vi "Parse Variant.vi"(8 "error in":errorcluster, 10 "Data":variant) -> (0 "error out":errorcluster, 1 "Types":T1[](array[typedef]), 2 "Data":string[](array[string]), 3 "Variants":variant[](array[variant]), 4 "Type (Name)":string[](array[string]))   [LabVIEW 2019, in "LV-Data.PGSQL.lvclass"]
uses:
  LV-Data.PGSQL.lvclass
  <vilib>/Utility/Data Type/Type Definitions/Data Type.ctl
  Typedefs/Errors--enum.ctl
  Typedefs/Time.Datatype--enum.ctl
  <vilib>/Utility/Data Type/NI_Data Type.lvlib
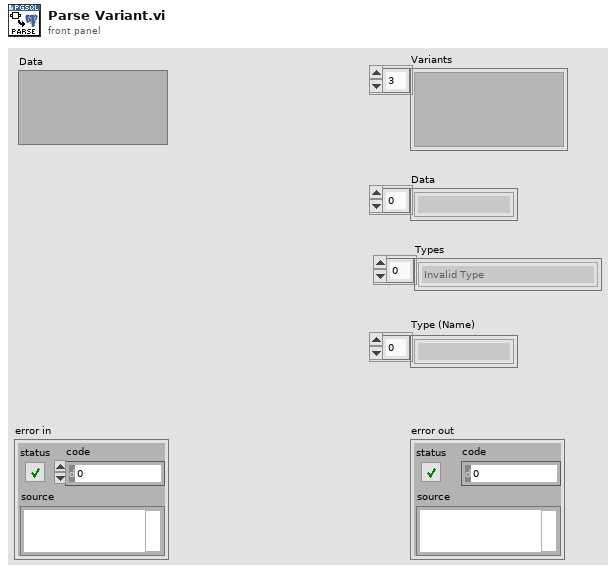
[diagram p1: front panel]
types:
  T1 = typedef "NI_Data Type.lvlib/Data Type.ctl" = enum8{"Invalid Type", "Void", "I8", "I16", "I32", "I64", "U8", "U16", "U32", "U64", "Single Float", "Double Float", "Extended Float", "Single Complex", "Double Complex", "Extended Complex", "Enum U8", "Enum U16", "Enum U32", "Enum U64", "Single Float With Unit", "Double Float With Unit", "Extended Float With Unit", "Single Complex with Unit", "Double Complex with Unit", "Extended Complex with Unit", "Boolean", "String", "Path", "Picture", "Tag", "Array", "Cluster", "Variant", "LV Variant", "Waveform", "Timestamp", "Digital Waveform", "Digital Data", "ExpressData", "Refnum", "External Data", "VI", "Poly VI", "LabVIEW Class Instance", "Fixed Point", "Set Collection", "Map Collection"}
  T2 = typedef "LV-Data.PGSQL.lvclass/Errors--enum.ctl" = enum16{"0: None", "5005: Path Type Not Supported", "5006: Number of Variables", "5007: Number of data points", "5008: Cannot write two data points", "5030: Start and End Times Identical", "5031: Input is not wholly", "5032: Undefined Timestamps", "5033: Bad path or paths", "5040: Invalid Instrument Name", "5050: Column can only hold string", "5051: Column can only hold bool", "5052: Column can only hold double", "5053: Column can only hold int"}
  T3 = typedef "LV-Data.PGSQL.lvclass/Time.Datatype--enum.ctl" = enum16{"timestamp without time zone", "timestamp with time zone"}
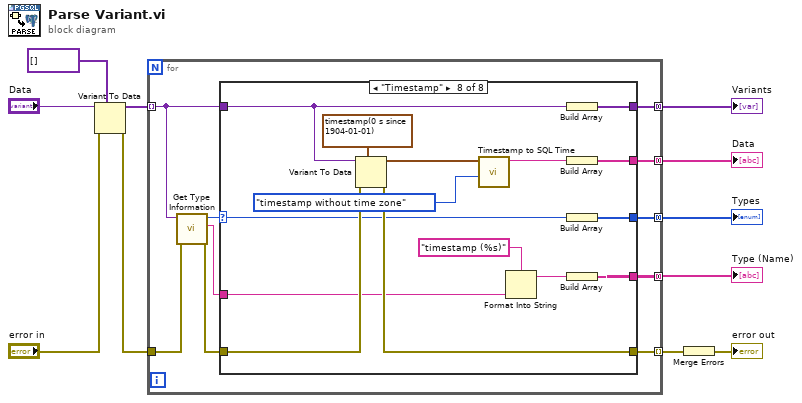
[diagram p0: block diagram]
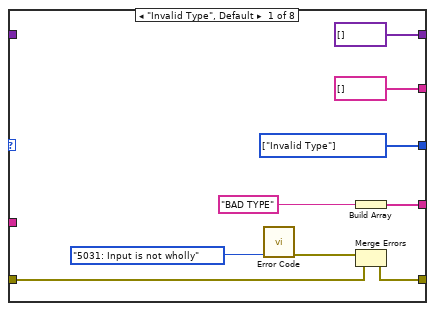
[diagram p2: hidden frame]
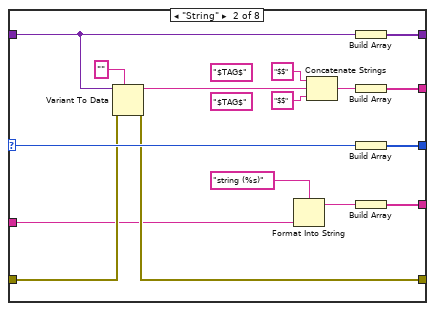
[diagram p3: hidden frame]
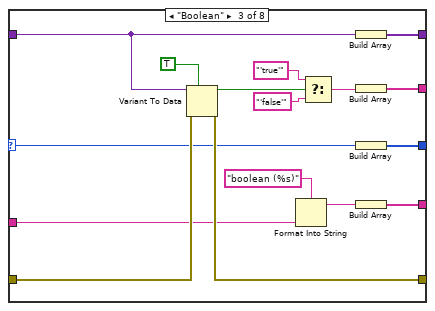
[diagram p4: hidden frame]
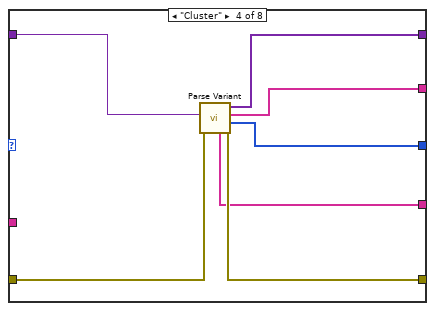
[diagram p5: hidden frame]
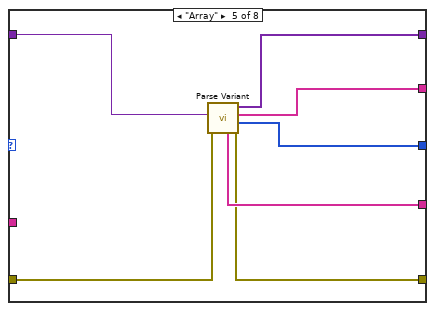
[diagram p6: hidden frame]
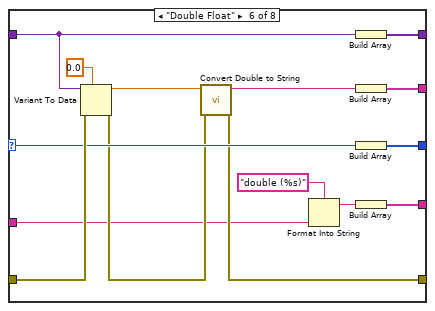
[diagram p7: hidden frame]
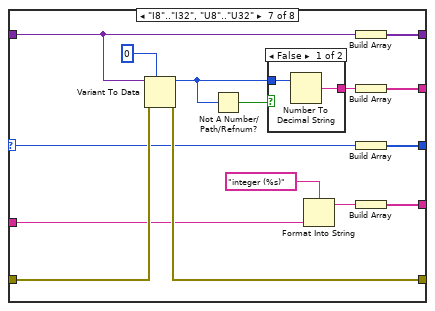
[diagram p8: hidden frame]
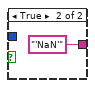
[diagram p9: hidden frame]
diagram:
  n1 = Variant To Data(error in="error in", type=variant[] [] ("Variants"), Variant="Data") -> (data=w2:variant[], error out=w3:errorcluster)
  n2 = for {
    tunnel: w2 -> [w16] mode=indexing
    tunnel: [w20] -> w11 mode=concatenating
    tunnel: [w19] -> w10 mode=concatenating
    tunnel: [w18] -> w9 mode=concatenating
    tunnel: [w13] -> w7 mode=indexing
    tunnel: w3 -> [w15]
    tunnel: [w17] -> w6 mode=concatenating
    n3 = call <vilib>:"Get Type Information.vi"("error in (no error)"=w15, "variant"=w16) -> ("error out"=w14:errorcluster, "name"=w12:string, "type"=w21:T1)  [unwired: 5 in, 2 out]
    n4 = case shown="\"Timestamp\"" w21 {
      selector: w21 -> [_ w36 w50 _ _ w83 w98 w118]
      tunnel: w16 -> [_ w39 w55 w69 w76 w86 w95 w117]
      tunnel: [string[] [] ("Strings") w41 w57 w64 w75 w89 w103 w122] -> w19
      tunnel: [w28 w40 w56 w65 w70 w90 w105 w124] -> w20
      tunnel: [variant[] [] ("Variants") w38 w54 w63 w71 w87 w104 w123] -> w18
      tunnel: [w27 w37 w53 w66 w74 w85 w101 w121] -> w17
      tunnel: w14 -> [w25 w35 w52 w68 w73 w84 w100 w120]
      tunnel: [w24 w34 w51 w67 w72 w80 w99 w119] -> w13
      tunnel: w12 -> [_ w32 w49 _ _ w78 w92 w112]
      frame "Invalid Type", Default {
        w28 = T1[] [enum."Invalid Type"] items=["Invalid Type", "Void", "I8", "I16", "I32", "I64", "U8", "U16", "U32", "U64", "Single Float", "Double Float", "Extended Float", "Single Complex", "Double Complex", "Extended Complex", "Enum U8", "Enum U16", "Enum U32", "Enum U64", "Single Float With Unit", "Double Float With Unit", "Extended Float With Unit", "Single Complex with Unit", "Double Complex with Unit", "Extended Complex with Unit", "Boolean", "String", "Path", "Picture", "Tag", "Array", "Cluster", "Variant", "LV Variant", "Waveform", "Timestamp", "Digital Waveform", "Digital Data", "ExpressData", "Refnum", "External Data", "VI", "Poly VI", "LabVIEW Class Instance", "Fixed Point", "Set Collection", "Map Collection"] ("Types")
        n5 = call "Error Code.vi"("Error code"=Errors--enum."5031: Input is not wholly") -> ("error out"=w22:errorcluster)  [unwired: 10 in]
        n6 = Build Array("BAD TYPE") -> (w27:string[])
        n7 = Merge Errors(w22, w25) -> (w24:errorcluster)
      }
      frame "String" {
        (unwired) "$TAG$" ("string")
        (unwired) "$TAG$" ("string")
        n8 = Variant To Data(error in=w35, type="", Variant=w39) -> (data=w45:string, error out=w34:errorcluster)
        n9 = Format Into String(format string="string (%s)", w32) -> (resulting string=w31:string)  [unwired: 2 in, 1 out]
        n10 = Concatenate Strings("$$" ("string"), w45, "$$" ("string")) -> (w42:string)
        n11 = Build Array(w39) -> (w38:variant[])
        n12 = Build Array(w42) -> (w41:string[])
        n13 = Build Array(w36) -> (w40:T1[])
        n14 = Build Array(w31) -> (w37:string[])
      }
      frame "Boolean" {
        n15 = Variant To Data(error in=w52, type=TRUE, Variant=w55) -> (data=w61:bool, error out=w51:errorcluster)
        n16 = Format Into String(format string="boolean (%s)", w49) -> (resulting string=w48:string)  [unwired: 2 in, 1 out]
        n17 = Select(t="'true'", s=w61, f="'false'") -> (s? t:f=w58:string)
        n18 = Build Array(w55) -> (w54:variant[])
        n19 = Build Array(w58) -> (w57:string[])
        n20 = Build Array(w50) -> (w56:T1[])
        n21 = Build Array(w48) -> (w53:string[])
      }
      frame "Cluster" {
        n22 = call "Parse Variant.vi"("error in"=w68, "Data"=w69) -> ("error out"=w67:errorcluster, "Types"=w65:T1[], "Data"=w64:string[], "Variants"=w63:variant[], "Type (Name)"=w66:string[])  [unwired: 5 in]
      }
      frame "Array" {
        n23 = call "Parse Variant.vi"("error in"=w73, "Data"=w76) -> ("error out"=w72:errorcluster, "Types"=w70:T1[], "Data"=w75:string[], "Variants"=w71:variant[], "Type (Name)"=w74:string[])  [unwired: 5 in]
      }
      frame "Double Float" {
        n24 = Variant To Data(error in=w84, type=0.0, Variant=w86) -> (data=w82:dbl, error out=w81:errorcluster)
        n25 = call "Convert Double to String.vi"("error in"=w81, "Numeric"=w82) -> ("error out"=w80:errorcluster, "PGSQL String"=w88:string)  [unwired: 8 in]
        n26 = Format Into String(format string="double (%s)", w78) -> (resulting string=w77:string)  [unwired: 2 in, 1 out]
        n27 = Build Array(w86) -> (w87:variant[])
        n28 = Build Array(w88) -> (w89:string[])
        n29 = Build Array(w83) -> (w90:T1[])
        n30 = Build Array(w77) -> (w85:string[])
      }
      frame "I8".."I32", "U8".."U32" {
        n31 = Variant To Data(error in=w100, type=0, Variant=w95) -> (data=w96:i32, error out=w99:errorcluster)
        n32 = Not A Number/Path/Refnum?(number/path/refnum=w96) -> (NaN/Path/Refnum?=w97:bool)
        n33 = case shown="False" w97 {
          tunnel: [w108 "'NaN'"] -> w102
          tunnel: w96 -> [w107 _]
          frame False {
            n34 = Number To Decimal String(number=w107) -> (decimal integer string=w108:string)  [unwired: 1 in]
          }
          frame True {
          }
        }
        n35 = Format Into String(format string="integer (%s)", w92) -> (resulting string=w93:string)  [unwired: 2 in, 1 out]
        n36 = Build Array(w95) -> (w104:variant[])
        n37 = Build Array(w102) -> (w103:string[])
        n38 = Build Array(w98) -> (w105:T1[])
        n39 = Build Array(w93) -> (w101:string[])
      }
      frame "Timestamp" {
        n40 = Variant To Data(error in=w120, type=timestamp(0 s since 1904-01-01) ("Time Stamp"), Variant=w117) -> (data=w116:timestamp, error out=w119:errorcluster)
        n41 = call "Timestamp to SQL Time.vi"("Time Datatype"=Time.Datatype--enum."timestamp without time zone", "Timestamp"=w116) -> ("date/time string"=w115:string)  [unwired: 9 in]
        n42 = Format Into String(format string="timestamp (%s)", w112) -> (resulting string=w113:string)  [unwired: 2 in, 1 out]
        n43 = Build Array(w117) -> (w123:variant[])
        n44 = Build Array(w115) -> (w122:string[])
        n45 = Build Array(w118) -> (w124:T1[])
        n46 = Build Array(w113) -> (w121:string[])
      }
    }
  }
  "Variants" <- w9
  "Types" <- w11
  "Data" <- w10
  "Type (Name)" <- w6
  n47 = Merge Errors(w7) -> (→"error out":errorcluster)
